vi "TargetsUI.vi"() -> ()   [LabVIEW 2019, in "Targets.lvclass"]
uses:
  Targets.lvclass
  <vilib>/NI/Configuration Framework/Node/NodeRef.ctl
  <vilib>/NI/Configuration Framework/Node/NISE_CEF_Node.lvclass
  <vilib>/NI/AMC/Message Queue.ctl
  <vilib>/NI/AMC/Message.ctl
  <vilib>/NI/Tools/Keyed Array/KeyedArray.ctl
  <vilib>/NI/Configuration Framework/Node/UserEventRef.ctl
  <vilib>/NI/Configuration Framework/Controls/EventCluster.ctl
  C:/Program Files (x86)/National Instruments/LabVIEW 2019/vi.lib/NI/Configuration Framework/Node/NISE_CEF_Node.lvclass
  <vilib>/NI/Configuration Framework/Node/NISE_CEF_Node.lvclass/NISE_CEF_Node.ctl
  Targets.lvclass/Targets.ctl
  Target/Target.lvclass
  Read Section Name.vi
  Write Section Name.vi
  <vilib>/NI/AMC/Create Single Message.vi
  <vilib>/NI/AMC/Update Message Routing Info.vi
  <vilib>/NI/AMC/Send Message.vi
  <vilib>/NI/AMC/AMC.lvlib
  Configuration Tool.lvlib
  <vilib>/NI/Tools/Keyed Array/Tools_KeyedArray.lvlib
  <vilib>/NI/Configuration Framework/NISE_CEF_TreeControl.lvlib
panel:
  in  "Main UI Tab":enum32{"Targets"}(tab)
  out "Targets Added to System Definition":i32(listbox)
  in  "Show Documentation":bool
  in  "user event":T1
  in  "main queue":T2
  out "Section Name":string
  in  "node ref":T3
  # "Supported Targets"
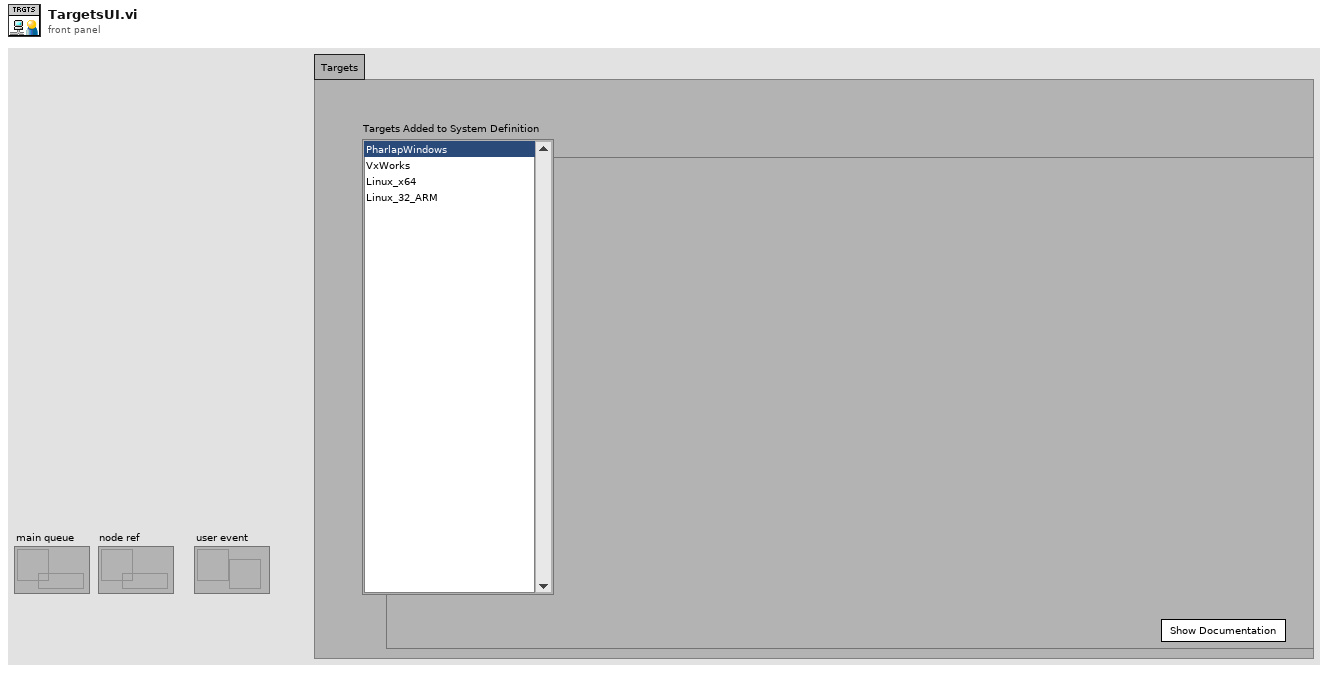
[diagram p1: front panel]
types:
  T1 = typedef "NISE_CEF_Node.lvclass/UserEventRef.ctl" = refnum<user-event>
  T2 = typedef "AMC.lvlib/Message Queue.ctl" = refnum<queue>
  T3 = typedef "NISE_CEF_Node.lvclass/NodeRef.ctl" = refnum<data-value>
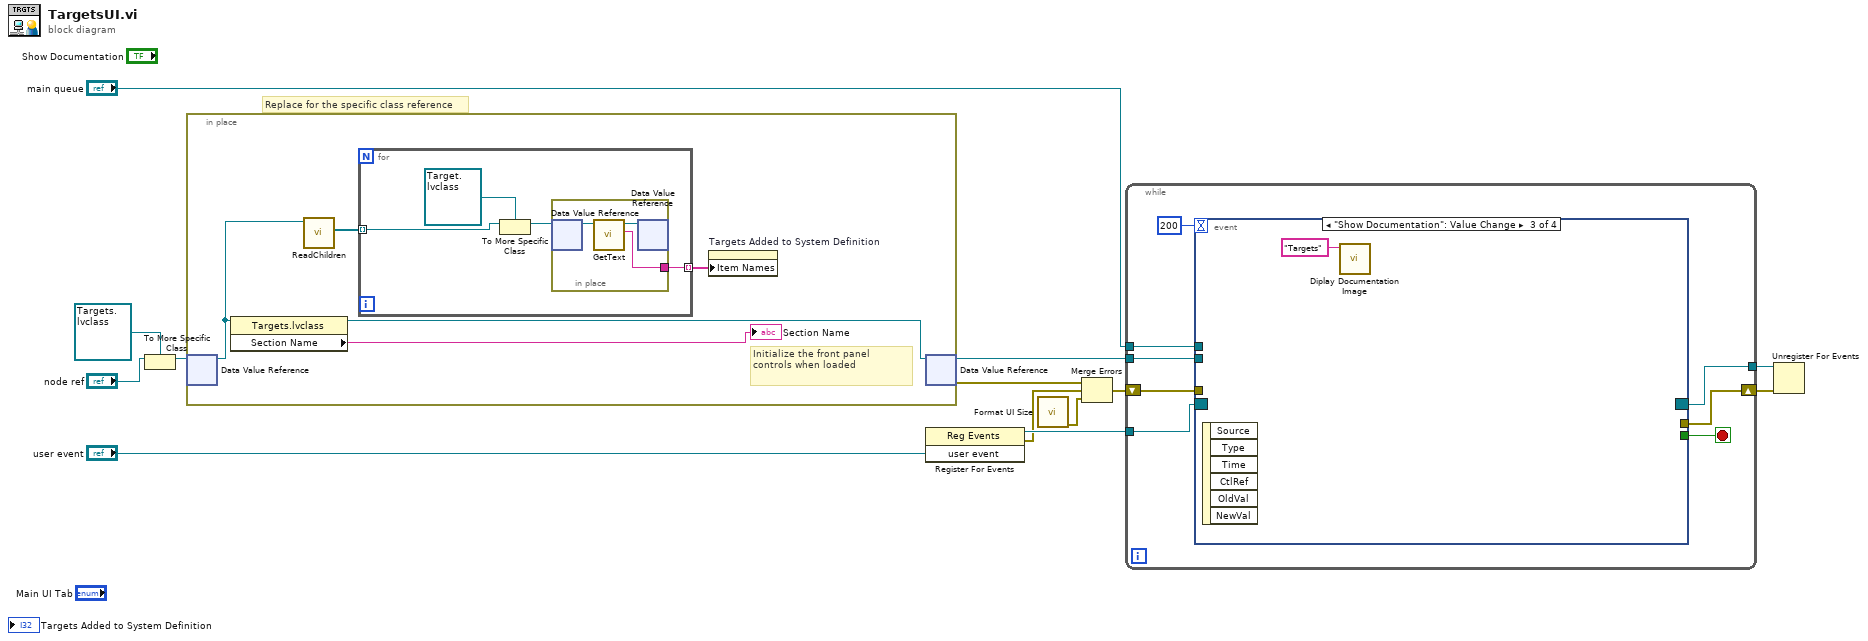
[diagram p0: block diagram]
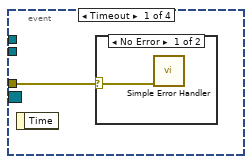
[diagram p2: hidden frame]
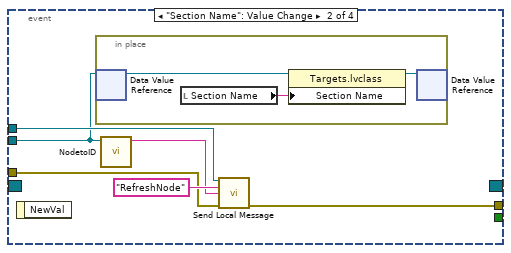
[diagram p4: hidden frame]
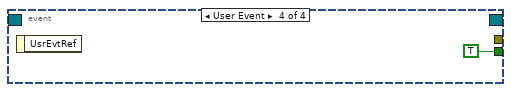
[diagram p5: hidden frame]
diagram:
  # "Replace for the specific class reference"
  n1 = To More Specific Class(target class=refnum<data-value> refnum ("data value reference"), reference="node ref") -> (specific class reference=w6:refnum<data-value>)  [unwired: 1 in, 1 out]
  n2 = in-place {
    # "Initialize the front panel controls when loaded"
    n3 = in-place-dvr #1(w6) -> (w17:refnum<class "Targets.lvclass">)  [unwired: 1 out]
    n4 = property class="Targets.lvclass"(reference=w17) -> (reference out=w16:refnum<class "Targets.lvclass">, "Section Name"=→"Section Name":string)  [unwired: 1 in, 1 out]
    n5 = call <vilib>:"ReadChildren.vi"("node in"=w17) -> ("output array"=w14:T3[])  [unwired: 8 in, 2 out]
    n6 = for {
      tunnel: [w22] -> w15 mode=indexing
      tunnel: w14 -> [w19] mode=indexing
      n7 = To More Specific Class(target class=refnum<data-value> refnum, reference=w19) -> (specific class reference=w20:refnum<data-value>)  [unwired: 1 in, 1 out]
      n8 = in-place {
        in-place-border: [w24] -> w22
        n9 = in-place-dvr #2(w20) -> (w25:refnum<class "Target.lvclass">)  [unwired: 1 out]
        n10 = call-dynamic "GetText.vi"("node in"=w25) -> ("text"=w24:string, "node out"=w23:refnum<class "Target.lvclass">)  [unwired: 6 in, 3 out]
        n11 = in-place-dvr #2(w23) -> ()  [unwired: 2 out]
      }
    }
    n12 = property on="Targets Added to System Definition" class="LstBox (strict)"("Item Names"=w15) -> ()  [unwired: 2 in, 2 out]
    n13 = in-place-dvr #1(w16) -> (w13:refnum<data-value>, w3:errorcluster)
  }
  n14 = register-events("user event") -> (reference out=w10:refnum<event-registration>, error out=w4:errorcluster)  [unwired: 2 in]
  n15 = call "Format UI Size.vi"() -> ("error out"=w1:errorcluster)  [unwired: 11 in]
  n16 = Merge Errors(w3, w4, w1) -> (w2:errorcluster)
  n17 = while {
    tunnel: w13 -> [w33]
    tunnel: "main queue" -> [w32]
    tunnel: w10 -> [w30]
    tunnel: [w29] -> w9
    shift-right: [w27] -> w8
    shift-left: w2 -> [w26]
    stop <- w28 stop-if-true
    n18 = event shown="[2] \"Show Documentation\": Value Change" {
      selector: w30 -> [_ _ _ _]
      dyn-events: [_ _ _ _] -> w29
      timeout: 200 -> [_ _ _ _]
      tunnel: w33 -> [_ w39 _ _]
      tunnel: w32 -> [_ w40 _ _]
      tunnel: [_ _ _ TRUE] -> w28
      tunnel: [_ w37 _ _] -> w27
      tunnel: w26 -> [w34 w36 _ _]
      event Timeout {
        n19 = event-data() -> ()  [unwired: 1 in, 1 out]
        n20 = case shown="No Error" w34 {
          selector: w34 -> [w35 _]
          frame No Error {
            n21 = call <vilib>:"Simple Error Handler.vi"("error in (no error)"=w35) -> ()  [unwired: 4 in, 5 out]
          }
          frame Error {
          }
        }
      }
      event "Section Name": Value Change {
        n22 = event-data() -> ()  [unwired: 1 in, 1 out]
        n23 = in-place {
          n24 = in-place-dvr #3(w39) -> (w44:refnum<class "Targets.lvclass">)  [unwired: 1 out]
          n25 = local read "Section Name"() -> (w42:string)
          n26 = property class="Targets.lvclass"(reference=w44, "Section Name"=w42) -> (reference out=w43:refnum<class "Targets.lvclass">)  [unwired: 1 in, 1 out]
          n27 = in-place-dvr #3(w43) -> ()  [unwired: 2 out]
        }
        n28 = call <vilib>:"NodetoID.vi"("node ref"=w39) -> ("ID"=w38:string)  [unwired: 9 in, 1 out]
        n29 = call <vilib>:"Send Local Message.vi"("message queue in"=w40, "message name"="RefreshNode" ("Message Name"), "message value"=w38, "error in"=w36) -> ("error out"=w37:errorcluster)  [unwired: 9 in, 2 out]
      }
      event "Show Documentation": Value Change {
        n30 = event-data() -> ()  [unwired: 1 in, 6 out]
        n31 = call "Diplay Documentation Image.vi"("Image Name"="Targets") -> ()  [unwired: 10 in, 1 out]
      }
      event User Event {
        n32 = event-data() -> ()  [unwired: 1 in, 1 out]
      }
    }
  }
  n33 = Unregister For Events(event registration refnum=w9, error in=w8) -> ()  [unwired: 1 out]
